vi "Read Motor Velocity Setpoints of Single Wheel.vi"(7 "wheel index":i32, 8 "error in (no error)":errorcluster, 11 "steering frame in":refnum<class "NI_Robotics_Steering Frame.lvclass">) -> (0 "error out":errorcluster, 1 "ccw motor angle setpoint (rad)":dbl, 2 "ccw motor velocity setpoint":dbl, 3 "steering frame out":refnum<class "NI_Robotics_Steering Frame.lvclass">, 4 "ccw caster motor velocity setpoint":dbl)   [LabVIEW 2017, in "NI_Robotics_Steering Frame.lvclass"]
uses:
  <vilib>/robotics/Steering/Steering Frame/NI_Robotics_Steering Frame.lvclass
  <vilib>/robotics/Steering/Steering Frame/NI_Robotics_Steering Frame.lvclass/NI_Robotics_Steering Frame.ctl
  <vilib>/robotics/Steering/Wheel/Get Motor Velocity Setpoint.vi
  <vilib>/robotics/Steering/Wheel/NI_Robotics_Wheel.lvclass
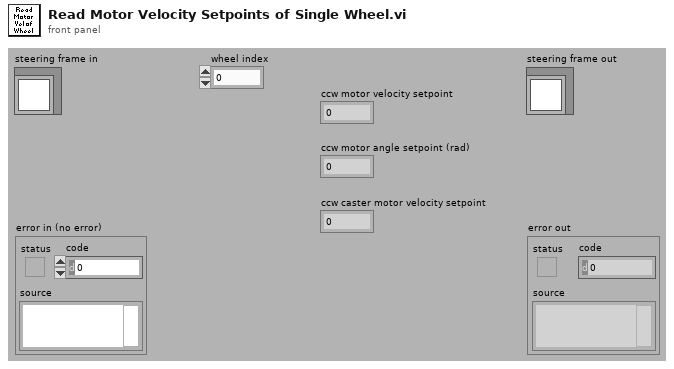
[diagram p1: front panel]
types:
  T1 = typedef "NI_Robotics_Steering Frame.lvclass/Wheel Orientation.ctl" = cluster{"wheel":refnum<class "NI_Robotics_Wheel.lvclass">, "x position":dbl, "y position":dbl, "frame angle (rad)":dbl}
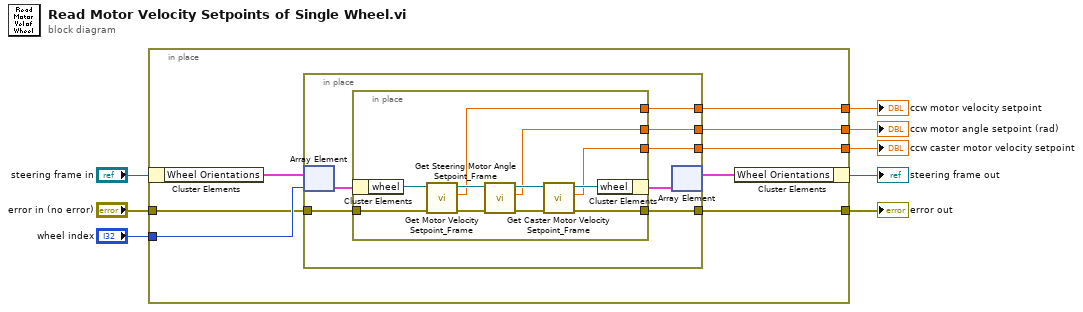
[diagram p0: block diagram]
diagram:
  n1 = in-place {
    in-place-border: "wheel index" -> [w16]
    in-place-border: "error in (no error)" -> [w15]
    in-place-border: [w12] -> w4
    in-place-border: [w11] -> w3
    in-place-border: [w10] -> w2
    in-place-border: [w9] -> w1
    n2 = in-place-cluster #1("steering frame in") -> ("Wheel Orientations"=w14:T1[])
    n3 = in-place {
      in-place-border: w15 -> [w23]
      in-place-border: [w20] -> w12
      in-place-border: [w19] -> w11
      in-place-border: [w18] -> w10
      in-place-border: [w17] -> w9
      n4 = in-place-array #2(w14, w16) -> (w22:T1)
      n5 = in-place {
        in-place-border: w23 -> [w30]
        in-place-border: [w27] -> w20
        in-place-border: [w26] -> w19
        in-place-border: [w25] -> w18
        in-place-border: [w24] -> w17
        n6 = in-place-cluster #3(w22) -> ("wheel"=w34:refnum<class "NI_Robotics_Wheel.lvclass">)
        n7 = call <vilib>:"Get Motor Velocity Setpoint_Frame.vi"("error in (no error)"=w30, "wheel in"=w34) -> ("error out"=w29:errorcluster, "ccw motor velocity setpoint"=w24:dbl, "wheel out"=w33:refnum<class "NI_Robotics_Wheel.lvclass">)  [unwired: 6 in, 1 out]
        n8 = call <vilib>:"Get Steering Motor Angle Setpoint_Frame.vi"("error in (no error)"=w29, "wheel in"=w33) -> ("error out"=w28:errorcluster, "ccw motor angle setpoint (rad)"=w25:dbl, "wheel out"=w32:refnum<class "NI_Robotics_Wheel.lvclass">)  [unwired: 6 in, 1 out]
        n9 = call <vilib>:"Get Caster Motor Velocity Setpoint_Frame.vi"("error in (no error)"=w28, "wheel in"=w32) -> ("error out"=w27:errorcluster, "ccw caster motor velocity setpoint"=w26:dbl, "wheel out"=w31:refnum<class "NI_Robotics_Wheel.lvclass">)  [unwired: 6 in, 1 out]
        n10 = in-place-cluster #3("wheel"=w31) -> (w21:T1)
      }
      n11 = in-place-array #2(w21) -> (w13:T1[])  [unwired: 1 out]
    }
    n12 = in-place-cluster #1("Wheel Orientations"=w13) -> (→"steering frame out":refnum<class "NI_Robotics_Steering Frame.lvclass">)
  }
  "error out" <- w4
  "ccw motor angle setpoint (rad)" <- w2
  "ccw caster motor velocity setpoint" <- w3
  "ccw motor velocity setpoint" <- w1
